vi "Configure Analog Gen FFT Chirp.vi"(4 "FFT Source (0: csA0FFT)":i32(ring) items=["A0 FFT", "A0 FFT2Ch", "A1 FFT", "A1 FFT2Ch"], 5 "Enable Waveform (T: Enable)":bool=TRUE, 6 "Enable Variable Sweep (T: Enable)":bool=TRUE, 7 "Enable EQ Output Modification (T: Enable)":bool=TRUE, 8 "error in (no error)":errorcluster, 9 "Amplitude (0 Vrms)":dbl, 10 "Channel (0: A)":i32(ring) items=["A", "B"], 11 "VISA resource name":refnum<visa-resource-name>) -> (0 "error out":errorcluster, 3 "VISA resource name out":refnum<visa-resource-name>)   [LabVIEW 2014, in "Stanford Research SR1.lvlib"]
doc: "Configures the attributes of the Analog Generator FFT Chirp."
uses:
  Stanford Research SR1.lvlib
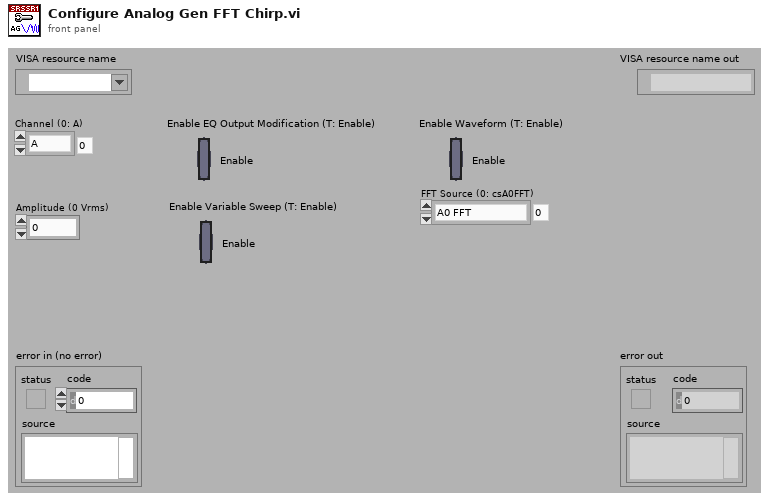
[diagram p1: front panel]
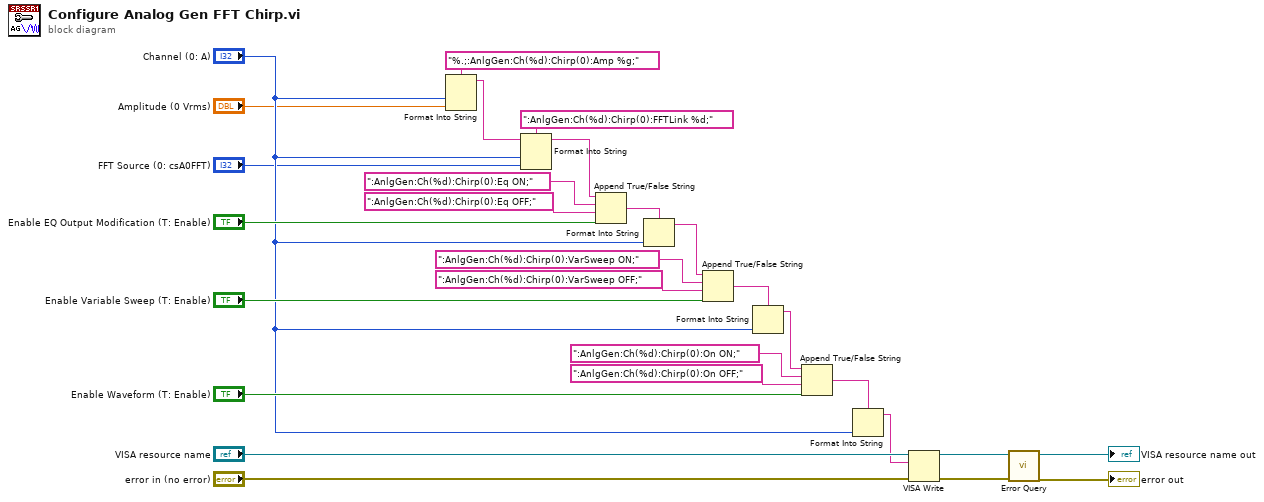
[diagram p0: block diagram]
diagram:
  n1 = Format Into String(format string="%.;:AnlgGen:Ch(%d):Chirp(0):Amp %g;", "Channel (0: A)", "Amplitude (0 Vrms)") -> (resulting string=w27:string)  [unwired: 2 in, 1 out]
  n2 = Format Into String(format string=":AnlgGen:Ch(%d):Chirp(0):FFTLink %d;", initial string=w27, "Channel (0: A)", "FFT Source (0: csA0FFT)") -> (resulting string=w25:string)  [unwired: 1 in, 1 out]
  n3 = Append True/False String(1:"Enable EQ Output Modification (T: Enable)", 2:":AnlgGen:Ch(%d):Chirp(0):Eq OFF;", 3:":AnlgGen:Ch(%d):Chirp(0):Eq ON;", 4:w25) -> (0:w7:string)
  n4 = Format Into String(format string=w7, "Channel (0: A)") -> (resulting string=w6:string)  [unwired: 2 in, 1 out]
  n5 = Append True/False String(1:"Enable Variable Sweep (T: Enable)", 2:":AnlgGen:Ch(%d):Chirp(0):VarSweep OFF;", 3:":AnlgGen:Ch(%d):Chirp(0):VarSweep ON;", 4:w6) -> (0:w5:string)
  n6 = Format Into String(format string=w5, "Channel (0: A)") -> (resulting string=w4:string)  [unwired: 2 in, 1 out]
  n7 = Append True/False String(1:"Enable Waveform (T: Enable)", 2:":AnlgGen:Ch(%d):Chirp(0):On OFF;", 3:":AnlgGen:Ch(%d):Chirp(0):On ON;", 4:w4) -> (0:w9:string)
  n8 = Format Into String(format string=w9, "Channel (0: A)") -> (resulting string=w8:string)  [unwired: 2 in, 1 out]
  n9 = VISA Write(VISA resource name="VISA resource name", write buffer=w8, error in (no error)="error in (no error)") -> (VISA resource name out=w13:refnum<visa-resource-name>, error out=w12:errorcluster)  [unwired: 1 out]
  n10 = call "Error Query.vi"("error in (no error)"=w12, "VISA resource name"=w13) -> ("error out"=→"error out":errorcluster, "VISA resource name out"=→"VISA resource name out":refnum<visa-resource-name>)  [unwired: 6 in, 2 out]
